vi "定时控制.vi"(9 "关闭时间（H）":u16, 10 "开启时间（H）":u16, 11 "控制模式":enum16{"手动", "自动"}(ring)) -> (3 "布尔":bool)   [LabVIEW 2016, in "random number.lvlib"]
uses:
  random number.lvlib
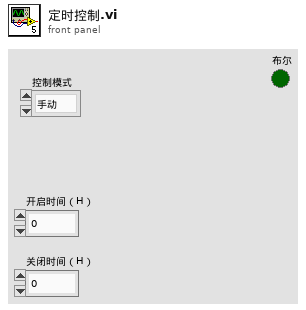
[diagram p1: front panel]
types:
  T1 = typedef "LVDateTimeRec.ctl" = cluster{"秒数的小数部分":dbl, "秒":i32, "分":i32, "时":i32, "日":i32, "月":i32, "年":i32, "天数（周）":i32, "天数（年）":i32, "DST":i32}
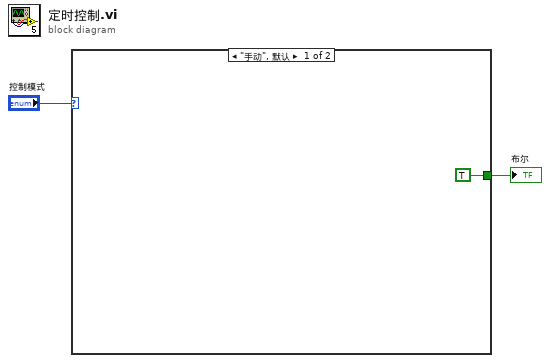
[diagram p0: block diagram]
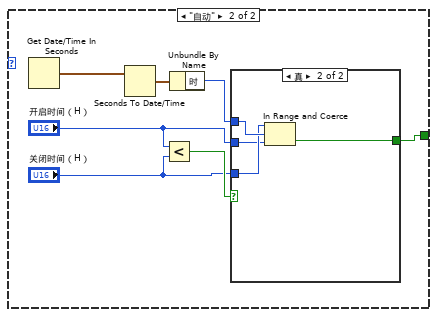
[diagram p2: hidden frame]
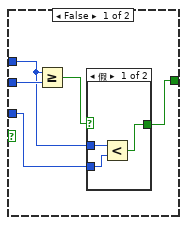
[diagram p3: hidden frame]
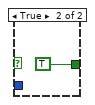
[diagram p4: hidden frame]
diagram:
  n1 = case shown="\"手动\", 默认" "控制模式" {
    tunnel: [TRUE w4] -> w2
    frame "手动", Default {
    }
    frame "自动" {
      n2 = Get Date/Time In Seconds() -> (seconds since 1Jan1904=w10:timestamp)
      n3 = Seconds To Date/Time(time stamp (now)=w10) -> (date time rec=w9:T1)  [unwired: 1 in]
      n4 = Less?(x="开启时间（H）", y="关闭时间（H）") -> (x < y?=w8:bool)
      n5 = Unbundle By Name(w9) -> ("时"=w7:i32)
      n6 = case shown="真" w8 {
        tunnel: w7 -> [w12 w23]
        tunnel: "关闭时间（H）" -> [w11 w22]
        tunnel: "开启时间（H）" -> [w15 w21]
        tunnel: [w13 w20] -> w4
        frame False {
          n7 = Greater Or Equal?(x=w12, y=w15) -> (x >= y?=w14:bool)
          n8 = case shown="假" w14 {
            tunnel: [w16 TRUE] -> w13
            tunnel: w12 -> [w18 _]
            tunnel: w11 -> [w17 _]
            frame False {
              n9 = Less?(x=w18, y=w17) -> (x < y?=w16:bool)
            }
            frame True {
            }
          }
        }
        frame True {
          n10 = In Range and Coerce(upper limit=w22, x=w23, lower limit=w21) -> (In Range?=w20:bool)  [unwired: 1 out]
        }
      }
    }
  }
  "布尔" <- w2
